vi "PRACTICA DE LED CON TIEMPO DE 500MS.vi"() -> ()   [LabVIEW 2017]
uses:
  <vilib>/MakerHub/LINX/LMH-LINX.lvlib
  <vilib>/MakerHub/LINX/Public/Utilities/Open Serial.vi
  <vilib>/MakerHub/LINX/Public/Peripherals/Digital/Digital Write 1 Chan.vi
  <vilib>/MakerHub/LINX/Public/Peripherals/Digital/Digital Read 1 Chan.vi
panel:
  in  "Serial Port":refnum<visa-resource-name>="N/A"
  in  "stop":bool
  out "Output Value":bool
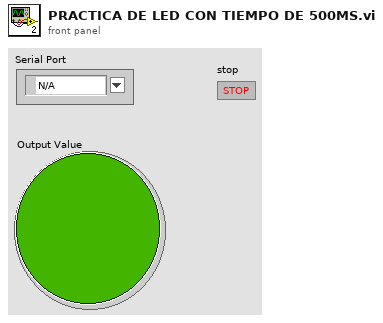
[diagram p1: front panel]
types:
  T1 = typedef "LMH-LINX.lvlib/LINX Ref.ctl" = cluster{"IO":T2, "Interface":T3, "LINX Device Config":T4}
  T2 = typedef "LMH-LINX.lvlib/Platform.ctl" = enum16{"Remote", "Local"}
  T3 = typedef "LMH-LINX.lvlib/Interface.ctl" = enum16{"Serial", "TCP"}
  T4 = typedef "LMH-LINX.lvlib/Device.lvlib/LINX Device Config.ctl" = cluster{"Interface":T3, "COM Port":refnum<visa-resource-name>, "TCP Configuration":T5, "Device Family":u8, "Device ID":u8, "Device Name":string, "TCP Ref":refnum<k5>, "Channels":T6}
  T5 = typedef "LMH-LINX.lvlib/Device.lvlib/TCP Config.ctl" = cluster{"IP Address":string, "Port":u16}
  T6 = typedef "LMH-LINX.lvlib/Channels.ctl" = cluster{"DI":u8[], "DO":u8[], "AI":u8[], "AO":u8[], "PWM":u8[], "QE":u8[], "UART":u8[], "I2C 2":u8[], "SPI":u8[], "CAN":u8[], "Servo":u8[], "AI Ref (V)":dbl, "AI Resolution (Bits)":u8, "AO Ref (V)":dbl, "AO Resolution (Bits)":u8}
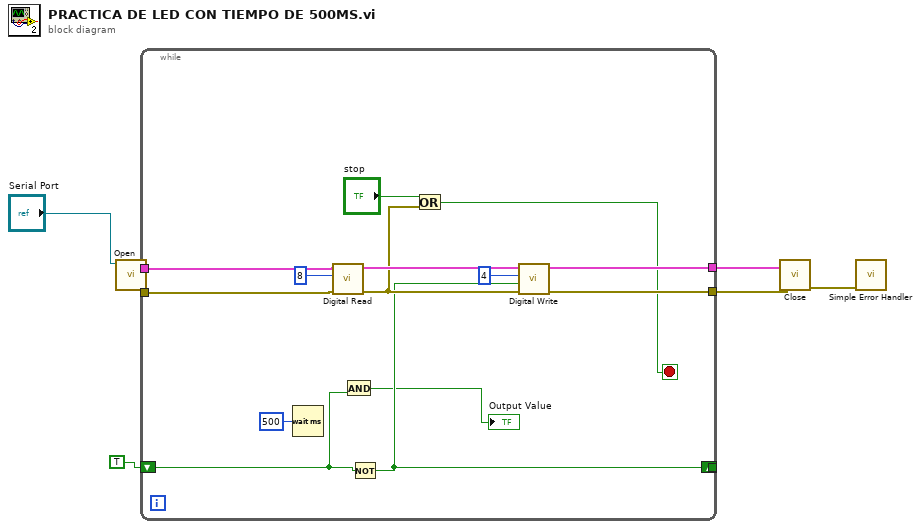
[diagram p0: block diagram]
diagram:
  n1 = call-poly <vilib>:"Open.vi"("Serial Port"="Serial Port") -> ("Error Out"=w7:errorcluster, "LINX Resource"=w4:T1)  [unwired: 8 in, 1 out]
  n2 = while {
    tunnel: w7 -> [w16]
    tunnel: [w21] -> w6
    tunnel: [w20] -> w5
    tunnel: w4 -> [w15]
    shift-right: [w12] -> _
    shift-left: TRUE -> [w9]
    tunnel: [w12] -> _
    stop <- w11 stop-if-true
    n3 = Wait (ms)(milliseconds to wait=u32 500) -> ()  [unwired: 1 out]
    n4 = call-poly <vilib>:"Digital Read.vi"("Error In"=w16, "DI Channel"=u8 8, "LINX Resource"=w15) -> ("Error Out"=w13:errorcluster, "LINX Resource"=w19:T1)  [unwired: 6 in, 1 out]
    n5 = And(y=w9) -> (x .and. y?=→"Output Value":bool)  [unwired: 1 in]
    n6 = Not(x=w9) -> (.not. x?=w12:bool)
    n7 = Or(x="stop", y=w13) -> (x .or. y?=w11:bool)
    n8 = call-poly <vilib>:"Digital Write.vi"("Error In"=w13, "Output Value"=w12, "DO Channel"=u8 4, "LINX Resource"=w19) -> ("Error Out"=w21:errorcluster, "LINX Resource"=w20:T1)  [unwired: 6 in]
  }
  n9 = call <vilib>:"Close.vi"("Error In"=w6, "LINX Resource"=w5) -> ("Error Out"=w3:errorcluster)  [unwired: 9 in]
  n10 = call <vilib>:"Simple Error Handler.vi"("error in (no error)"=w3) -> ()  [unwired: 4 in, 5 out]
